vi "FirstCode.vi"() -> ()   [LabVIEW 2015]
uses:
  <vilib>/myRIO/Instrument Drivers/Onboard IO/PWM/typedefs/PWM Reference.ctl
  <vilib>/myRIO/Common/Instrument Driver Framework/Utilities/typedefs/myRIO Generic Hardware Reference.ctl
  <vilib>/myRIO/Common/Instrument Driver Framework/Utilities/typedefs/Hardware Version Enum.ctl
  <vilib>/myRIO/Common/Instrument Driver Framework/Utilities/typedefs/myRIO v1.0 Reference.ctl
  <vilib>/myRIO/Common/Instrument Driver Framework/Utilities/typedefs/Generic FPGA Reference.ctl
  <vilib>/myRIO/Common/Instrument Driver Framework/myRIO v1.0/PWM/typedefs/PWM Channels Enum.ctl
  <vilib>/myRIO/Instrument Drivers/Onboard IO/PWM/typedefs/PWM Configuration.ctl
  <vilib>/userdefined/High Color/nirio_resource_hc.ctl
  <vilib>/myRIO/Instrument Drivers/Onboard IO/DIO/typedefs/DIO Reference.ctl
  <vilib>/myRIO/Common/Instrument Driver Framework/myRIO v1.0/DIO/typedefs/DIO Channels List.ctl
  <vilib>/myRIO/Common/Instrument Driver Framework/myRIO v1.0/DIO/typedefs/DIO Channels Enum.ctl
  <vilib>/myRIO/Common/Instrument Driver Framework/myRIO v1.0/PWM/vis/myRIO v1.1 Open PWM.vi
  <vilib>/myRIO/Common/Instrument Driver Framework/Utilities/vis/Is FPGA Ref Available.vi
  <vilib>/myRIO/Common/Instrument Driver Framework/myRIO v1.0/DIO/vis/myRIO v1.1 Open DIO.vi
  <vilib>/myRIO/Instrument Drivers/Onboard IO/DIO/vis/Read.vi
  <vilib>/myRIO/Instrument Drivers/Onboard IO/DIO/vis/Write.vi
  <vilib>/myRIO/Common/Instrument Driver Framework/Utilities/vis/Validate Channels.vi
  <vilib>/myRIO/Common/Instrument Driver Framework/myRIO v1.0/PWM/vis/myRIO v1.0 Reserve PWM.vi
  <vilib>/myRIO/Instrument Drivers/Onboard IO/PWM/vis/Set Duty Cycle and Frequency.vi
  <vilib>/myRIO/Common/Instrument Driver Framework/myRIO v1.0/DIO/vis/myRIO v1.0 Reserve DIO.vi
  <vilib>/myRIO/Common/Instrument Driver Framework/myRIO v1.0/PWM/vis/myRIO v1.0 Close PWM.vi
  <vilib>/myRIO/Common/Instrument Driver Framework/myRIO v1.0/UART/vis/myRIO v1.0 Close UART.vi
  <vilib>/myRIO/Common/Instrument Driver Framework/myRIO v1.0/PWM/vis/myRIO v1.0 Build MUX Configuration PWM.vi
  <vilib>/myRIO/Common/Instrument Driver Framework/myRIO v1.0/Resource Manager/vis/myRIO v1.0 Reserve Channel List.vi
  <vilib>/myRIO/Common/Instrument Driver Framework/myRIO v1.0/DIO/vis/myRIO v1.0 Build MUX Configuration DIO.vi
  <vilib>/myRIO/Common/Instrument Driver Framework/myRIO v1.0/PWM/vis/myRIO v1.0 Unreserve PWM.vi
  <vilib>/myRIO/Common/Instrument Driver Framework/myRIO v1.0/Resource Manager/vis/myRIO v1.0 Create Configuration List.vi
  <vilib>/myRIO/Common/Instrument Driver Framework/myRIO v1.0/Resource Manager/vis/myRIO v1.0 Reserve Channel.vi
  <vilib>/myRIO/Common/Instrument Driver Framework/myRIO v1.0/Resource Manager/vis/myRIO v1.0 Unreserve Channel.vi
  <vilib>/myRIO/Common/Instrument Driver Framework/myRIO v1.0/Resource Manager/vis/myRIO v1.0 Unreserve Channel List.vi
  <vilib>/myRIO/Common/Instrument Driver Framework/myRIO v1.0/Resource Manager/vis/myRIO v1.0 Build Mutex Name.vi
  <vilib>/Utility/VariantDataType/GetNumericInfo.vi
  <vilib>/Utility/error.llb/Error Cluster From Error Code.vi
  <vilib>/myRIO/Common/Instrument Driver Framework/myRIO v1.0/myRIO v1.1 Open.vi
  <vilib>/myRIO/Common/Instrument Driver Framework/Utilities/vis/IO Manager.vi
  <vilib>/myRIO/Common/Instrument Driver Framework/Utilities/vis/Configuration Manager.vi
  <vilib>/myRIO/Common/Instrument Driver Framework/myRIO v1.0/Resource Manager/vis/myRIO v1.0 Configure IO.vi
  <vilib>/myRIO/Common/Instrument Driver Framework/myRIO v1.0/myRIO v1.0 Close.vi
  <vilib>/myRIO/Common/Instrument Driver Framework/myRIO v1.0/PWM/vis/myRIO v1.0 Write PWM.vi
  <vilib>/myRIO/Common/Instrument Driver Framework/myRIO v1.0/DIO/vis/myRIO v1.0 Write DIO.vi
  <vilib>/myRIO/Common/Instrument Driver Framework/myRIO v1.0/DIO/vis/myRIO v1.0 Read DIO.vi
  <vilib>/myRIO/Common/Instrument Driver Framework/myRIO v1.0/PWM/vis/myRIO v1.0 Shutdown PWM.vi
  <vilib>/myRIO/Common/Instrument Driver Framework/Utilities/vis/FPGA Ref Manager.vi
  <vilib>/myRIO/Common/Instrument Driver Framework/myRIO v1.0/myRIO v1.0 Reset FPGA.vi
  <vilib>/myRIO/Common/Instrument Driver Framework/myRIO v1.0/IRQ/vis/myRIO v1.0 IRQ Info FGV.vi
  <vilib>/myRIO/Common/Instrument Driver Framework/myRIO v1.0/IRQ/vis/myRIO v1.0 Timer IRQ Info FGV.vi
  <vilib>/myRIO/Common/Instrument Driver Framework/myRIO v1.0/IRQ/vis/myRIO v1.0 ISR Agent.vi
  <vilib>/myRIO/Instrument Drivers/Onboard IO/PWM/vis/myRIO PWM Open.xnode
  <vilib>/myRIO/Express VI/Onboard Devices/LED/LED Express VI.xnode
  <vilib>/myRIO/Instrument Drivers/Onboard IO/DIO/vis/myRIO DIO Open.xnode
  <vilib>/myRIO/Express VI/Onboard IO/DI/DI Express VI.xnode
  <vilib>/myRIO/Instrument Drivers/Onboard IO/PWM/PWM.lvlib
  <vilib>/myRIO/Instrument Drivers/Onboard IO/DIO/DIO.lvlib
  <vilib>/myRIO/Instrument Drivers/Utilities/Utilities.lvlib
panel:
  out "Sensor Pin":T1
  out "Gripper Pin":T1
  out "Pour Pin":T1
  in  "Pour":bool
  out "Information":string="Pour"
  out "Counter":dbl=1.0
  out "New Duty Cycle":dbl=nan
  in  "Stop [ESC]":bool
  in  "Sensor":bool
  in  "Gripper":bool
  out "Water Detected":bool
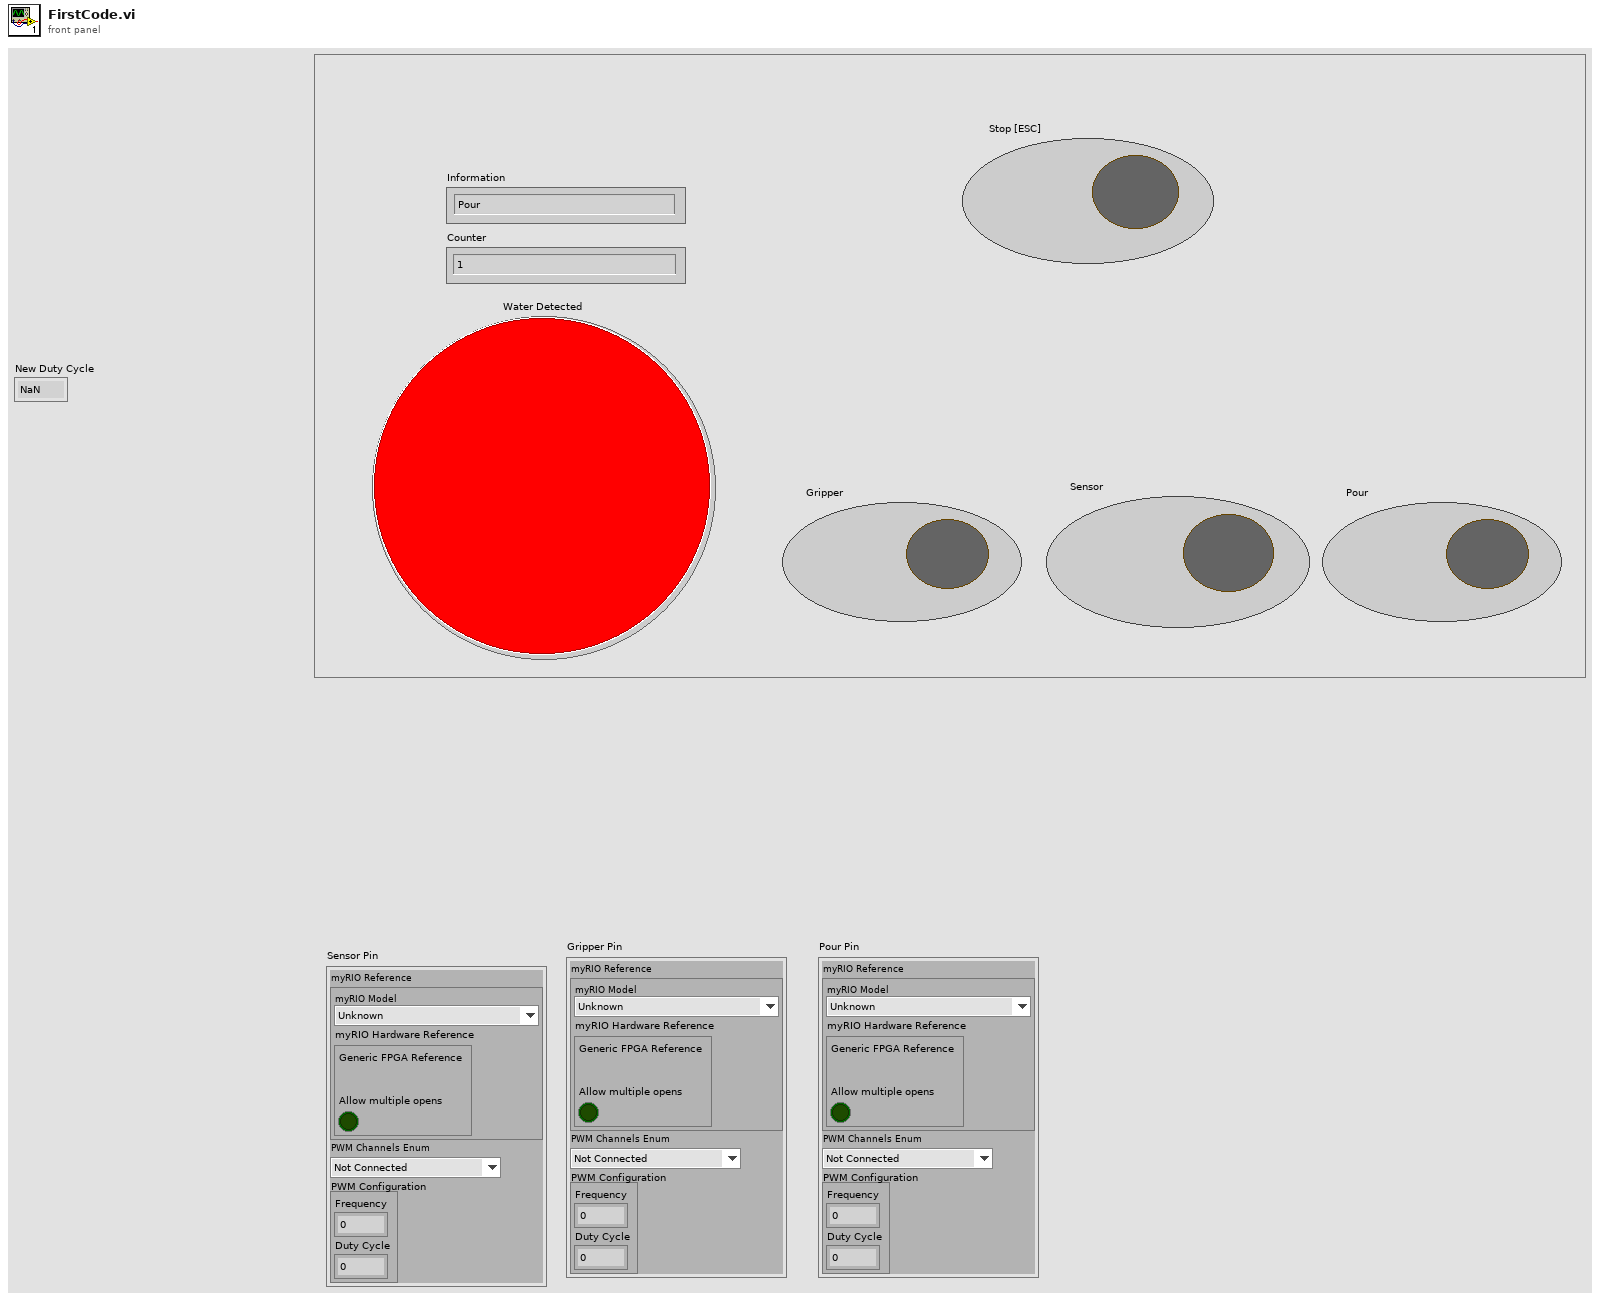
[diagram p1: front panel]
types:
  T1 = typedef "PWM.lvlib/PWM Reference.ctl" = cluster{"myRIO Reference":T2, "PWM Channels Enum":T6, "PWM Configuration":T7}
  T2 = typedef "myRIO Generic Hardware Reference.ctl" = cluster{"myRIO Model":T3, "myRIO Hardware Reference":T4}
  T3 = typedef "Hardware Version Enum.ctl" = enum16{"Unknown", "myRIO-1900", "myRIO-1950", "roboRIO"}
  T4 = typedef "myRIO v1.0 Reference.ctl" = cluster{"Generic FPGA Reference":T5, "Allow multiple opens":bool}
  T5 = typedef "Generic FPGA Reference.ctl" = refnum<k20>
  T6 = typedef "PWM Channels Enum.ctl" = enum16{"Not Connected", "C/PWM0", "C/PWM1", "A/PWM0", "A/PWM1", "A/PWM2", "B/PWM0", "B/PWM1", "B/PWM2", "PWM/PWM0", "PWM/PWM1", "PWM/PWM2", "PWM/PWM3", "PWM/PWM4", "PWM/PWM5", "PWM/PWM6", "PWM/PWM7", "PWM/PWM8", "PWM/PWM9"}
  T7 = typedef "PWM.lvlib/PWM Configuration.ctl" = cluster{"Frequency":dbl, "Duty Cycle":dbl}
  T8 = typedef "nirio_resource_hc.ctl" = tag
  T9 = typedef "DIO.lvlib/DIO Reference.ctl" = cluster{"myRIO Reference":T2, "DIO Channels List":T10}
  T10 = typedef "DIO Channels List.ctl" = T11[]
  T11 = typedef "DIO Channels Enum.ctl" = enum16{"Not Connected", "C/DIO0", "C/DIO1", "C/DIO2", "C/DIO3", "C/DIO4", "C/DIO5", "C/DIO6", "C/DIO7", "A/DIO0", "A/DIO1", "A/DIO2", "A/DIO3", "A/DIO4", "A/DIO5", "A/DIO6", "A/DIO7", "A/DIO8", "A/DIO9", "A/DIO10", "A/DIO11", "A/DIO12", "A/DIO13", "A/DIO14", "A/DIO15", "B/DIO0", "B/DIO1", "B/DIO2", "B/DIO3", "B/DIO4", "B/DIO5", "B/DIO6", "B/DIO7", "B/DIO8", "B/DIO9", "B/DIO10", "B/DIO11", "B/DIO12", "B/DIO13", "B/DIO14", "B/DIO15", "LED0", "LED1", "LED2", "LED3", "Button0", "DIO/DIO0", "DIO/DIO1", "DIO/DIO2", "DIO/DIO3", "DIO/DIO4", "DIO/DIO5", "DIO/DIO6", "DIO/DIO7", "DIO/DIO8", "DIO/DIO9", "SPI/CS0", "SPI/CS1", "SPI/CS2", "SPI/CS3", "LED RADIO (Green)", "LED RADIO (Red)", "LED COMM (Green)", "LED COMM (Red)", "LED MODE (Green)", "LED MODE (Red)"}
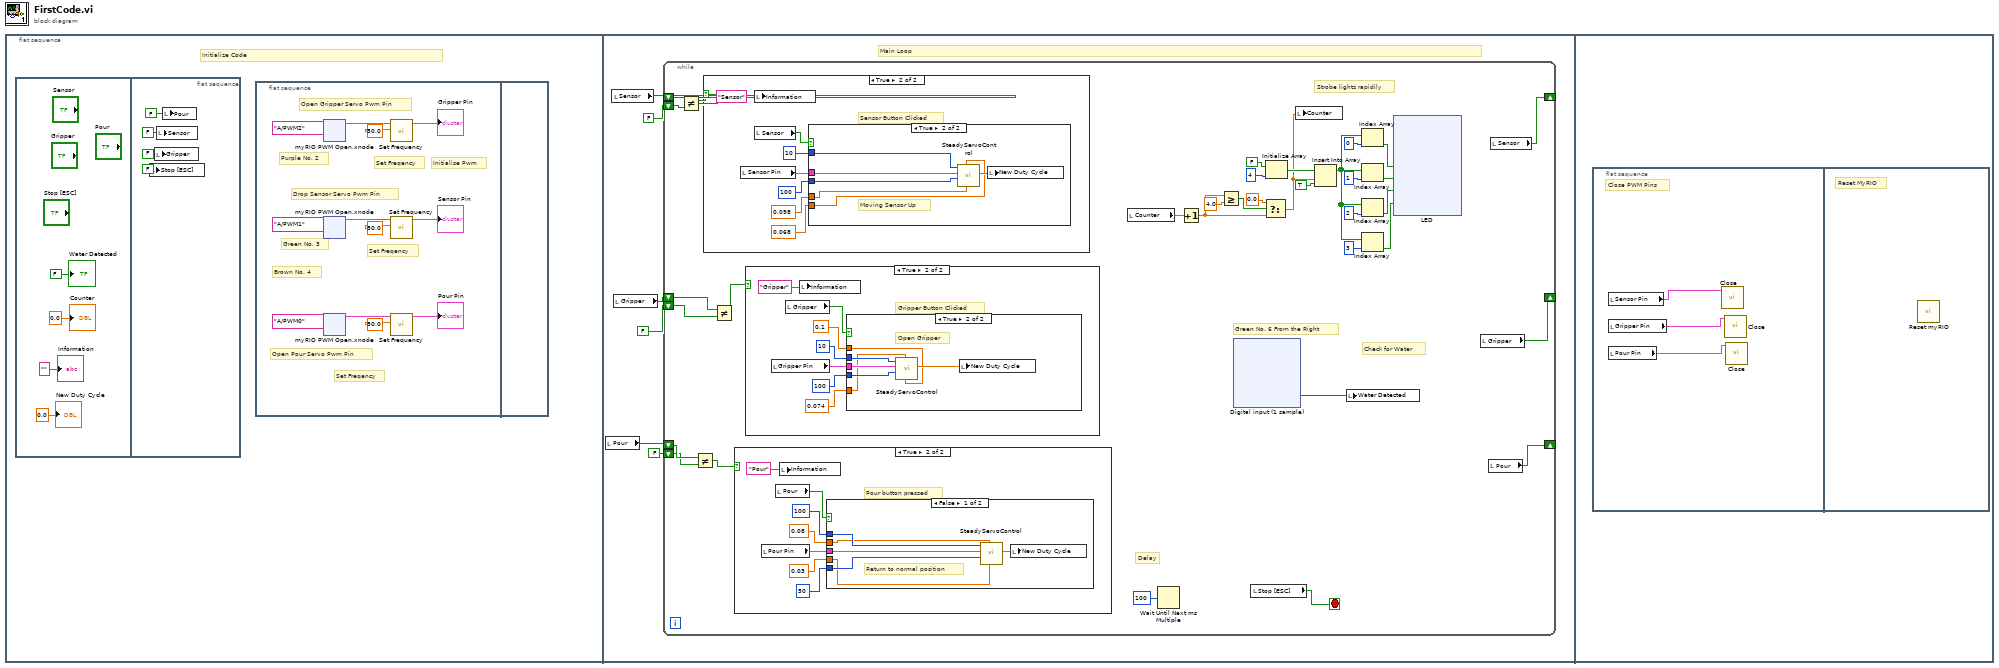
[diagram p0: block diagram]
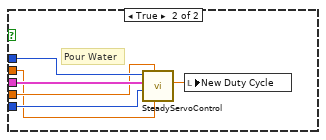
[diagram p3: hidden frame]
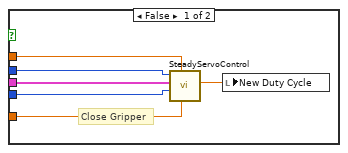
[diagram p5: hidden frame]
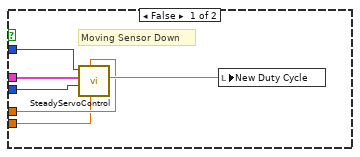
[diagram p7: hidden frame]
diagram:
  n1 = flat-sequence {
    frame #0 {
      # "Initialize Code"
      n2 = flat-sequence {
        frame #0 {
          "Water Detected" <- FALSE ("Water Detected")
          "Counter" <- 0.0 ("Counter")
          "Information" <- "" ("Information")
          "New Duty Cycle" <- 0.0 ("New Duty Cycle")
        }
        frame #1 {
          n3 = local write "Stop [ESC]"(FALSE ("Pour")) -> ()
          n4 = local write "Gripper"(FALSE ("Pour")) -> ()
          n5 = local write "Sensor"(FALSE ("Pour")) -> ()
          n6 = local write "Pour"(FALSE ("Pour")) -> ()
        }
      }
      n7 = flat-sequence {
        frame #0 {
          # "Green No. 3"
          # "Set Freqency"
          # "Drop Sensor Servo Pwm Pin"
          # "Initialise Pwm"
          # "Purple No. 2"
          # "Set Freqency"
          # "Open Gripper Servo Pwm Pin"
          # "Set Freqency"
          # "Brown No. 4"
          # "Open Pour Servo Pwm Pin"
          n8 = xnode "myRIO PWM Open.xnode"("Channel Name"=tag "A/PWM2") -> ("PWM Ref Out"=w7:T1)  [unwired: 2 in, 1 out]
          n9 = xnode "myRIO PWM Open.xnode"("Channel Name"=tag "A/PWM1") -> ("PWM Ref Out"=w2:T1)  [unwired: 2 in, 1 out]
          n10 = xnode "myRIO PWM Open.xnode"("Channel Name"=tag "A/PWM0") -> ("PWM Ref Out"=w10:T1)  [unwired: 2 in, 1 out]
          n11 = call <vilib>:"Set Frequency.vi"("Frequency [Hz]"=50.0, "PWM Ref In"=w7) -> ("PWM Ref Out"=→"Gripper Pin":T1)  [unwired: 7 in, 1 out]
          n12 = call <vilib>:"Set Frequency.vi"("Frequency [Hz]"=50.0, "PWM Ref In"=w2) -> ("PWM Ref Out"=→"Sensor Pin":T1)  [unwired: 7 in, 1 out]
          n13 = call <vilib>:"Set Frequency.vi"("Frequency [Hz]"=50.0, "PWM Ref In"=w10) -> ("PWM Ref Out"=→"Pour Pin":T1)  [unwired: 7 in, 1 out]
        }
        frame #1 {
        }
      }
    }
    frame #1 {
      # "Main Loop"
      n14 = local read "Pour"() -> (w70:bool)
      n15 = local read "Sensor"() -> (w74:bool)
      n16 = local read "Gripper"() -> (w72:bool)
      n17 = while {
        shift-right: [w108] -> _
        shift-left: w74 -> [w75]
        shift-left: FALSE ("Sensor") -> [w107]
        shift-right: [w105] -> _
        shift-left: w72 -> [w103]
        shift-left: FALSE ("Gripper") -> [w102]
        shift-right: [w76] -> _
        shift-left: w70 -> [w78]
        shift-left: FALSE ("Pour") -> [w77]
        stop <- w101 stop-if-true
        # "Delay"
        # "Check for Water"
        # "Strobe lights rapidily"
        # "Green No. 6 From the Right"
        n18 = Not Equal?(x=w75, y=w107) -> (x != y?=w106:bool)
        n19 = Not Equal?(x=w78, y=w77) -> (x != y?=w79:bool)
        n20 = case shown="True" w106 {
          frame False {
          }
          frame True {
            # "Sensor Button Clicked"
            n21 = local read "Sensor Pin"() -> (w222:T1)
            n22 = local write "Information"("Sensor" ("Information")) -> ()
            n23 = local read "Sensor"() -> (w225:bool)
            n24 = case shown="True" w225 {
              tunnel: u32 10 ("Wait Time") -> [w230 w237]
              tunnel: 100 ("Steps") -> [w229 w236]
              tunnel: w222 -> [w231 w235]
              tunnel: 0.098 ("t") -> [w228 w233]
              tunnel: 0.068 ("f") -> [w227 w234]
              frame False {
                # "Moving Sensor Down"
                n25 = call "SteadyServoControl.vi"("New Duty Cycle"=w227, "Prev Duty Cycle"=w228, "Steps"=w229, "PWM Ref Out in"=w231, "Wait Time"=w230) -> ("Numeric"=w232:dbl)  [unwired: 5 in, 1 out]
                n26 = local write "New Duty Cycle"(w232) -> ()
              }
              frame True {
                # "Moving Sensor Up"
                n27 = call "SteadyServoControl.vi"("New Duty Cycle"=w233, "Prev Duty Cycle"=w234, "Steps"=w236, "PWM Ref Out in"=w235, "Wait Time"=w237) -> ("Numeric"=w238:dbl)  [unwired: 5 in, 1 out]
                n28 = local write "New Duty Cycle"(w238) -> ()
              }
            }
          }
        }
        n29 = Not Equal?(x=w103, y=w102) -> (x != y?=w104:bool)
        n30 = case shown="True" w79 {
          frame False {
          }
          frame True {
            # "Pour button pressed"
            n31 = local read "Pour Pin"() -> (w113:T1)
            n32 = local read "Pour"() -> (w114:bool)
            n33 = local write "Information"("Pour" ("Information")) -> ()
            n34 = case shown="False" w114 {
              tunnel: w113 -> [w120 w127]
              tunnel: 50 ("Steps") -> [w118 w125]
              tunnel: u32 100 ("Wait Time") -> [w119 w124]
              tunnel: 0.03 ("Prev Duty Cycle") -> [w117 w123]
              tunnel: 0.08 ("New Duty Cycle") -> [w116 w122]
              frame False {
                # "Return to normal position"
                n35 = call "SteadyServoControl.vi"("New Duty Cycle"=w117, "Prev Duty Cycle"=w116, "Steps"=w118, "PWM Ref Out in"=w120, "Wait Time"=w119) -> ("Numeric"=w121:dbl)  [unwired: 5 in, 1 out]
                n36 = local write "New Duty Cycle"(w121) -> ()
              }
              frame True {
                # "Pour Water"
                n37 = call "SteadyServoControl.vi"("New Duty Cycle"=w122, "Prev Duty Cycle"=w123, "Steps"=w125, "PWM Ref Out in"=w127, "Wait Time"=w124) -> ("Numeric"=w126:dbl)  [unwired: 5 in, 1 out]
                n38 = local write "New Duty Cycle"(w126) -> ()
              }
            }
          }
        }
        n39 = case shown="True" w104 {
          frame False {
          }
          frame True {
            # "Gripper Button Clicked"
            n40 = local read "Gripper Pin"() -> (w205:T1)
            n41 = local read "Gripper"() -> (w206:bool)
            n42 = local write "Information"("Gripper" ("Information")) -> ()
            n43 = case shown="True" w206 {
              tunnel: w205 -> [w212 w216]
              tunnel: u32 10 ("Wait Time") -> [w211 w218]
              tunnel: 100 ("Steps") -> [w210 w217]
              tunnel: 0.074 ("Prev Duty Cycle") -> [w209 w215]
              tunnel: 0.1 ("New Duty Cycle") -> [w208 w214]
              frame False {
                # "Close Gripper"
                n44 = call "SteadyServoControl.vi"("New Duty Cycle"=w209, "Prev Duty Cycle"=w208, "Steps"=w210, "PWM Ref Out in"=w212, "Wait Time"=w211) -> ("Numeric"=w213:dbl)  [unwired: 5 in, 1 out]
                n45 = local write "New Duty Cycle"(w213) -> ()
              }
              frame True {
                # "Open Gripper"
                n46 = call "SteadyServoControl.vi"("New Duty Cycle"=w214, "Prev Duty Cycle"=w215, "Steps"=w217, "PWM Ref Out in"=w216, "Wait Time"=w218) -> ("Numeric"=w219:dbl)  [unwired: 5 in, 1 out]
                n47 = local write "New Duty Cycle"(w219) -> ()
              }
            }
          }
        }
        n48 = local read "Counter"() -> (w80:dbl)
        n49 = Wait Until Next ms Multiple(millisecond multiple=u32 100) -> ()  [unwired: 1 out]
        n50 = Increment(x=w80) -> (x+1=w95:dbl)
        n51 = Greater Or Equal?(x=w95, y=4.0) -> (x >= y?=w97:bool)
        n52 = xnode "Digital input (1 sample)"() -> ("A/DIO0 (Pin 11)"=w100:bool)  [unwired: 1 in, 1 out]
        n53 = local read "Stop [ESC]"() -> (w101:bool)
        n54 = Select(t=0.0, s=w97, f=w95) -> (s? t:f=w81:dbl)
        n55 = Initialize Array(FALSE, 4 ("dimension size")) -> (w84:bool[])
        n56 = local write "Counter"(w81) -> ()
        n57 = Insert Into Array(array=w84, index=w81, new element=TRUE ("new element/subarray")) -> (w83:bool[])
        n58 = local write "Water Detected"(w100) -> ()
        n59 = Index Array(array=w83, index=0) -> (element=w93:bool)
        n60 = Index Array(array=w83, index=1) -> (element=w87:bool)
        n61 = Index Array(array=w83, index=2) -> (element=w86:bool)
        n62 = Index Array(array=w83, index=3) -> (element=w85:bool)
        n63 = xnode "LED"("LED0"=w93, "LED1"=w87, "LED2"=w86, "LED3"=w85) -> ()  [unwired: 1 in, 1 out]
        n64 = local read "Gripper"() -> (w105:bool)
        n65 = local read "Pour"() -> (w76:bool)
        n66 = local read "Sensor"() -> (w108:bool)
      }
    }
    frame #2 {
      n67 = flat-sequence {
        frame #0 {
          # "Close PWM Pins"
          n68 = local read "Sensor Pin"() -> (w239:T1)
          n69 = local read "Gripper Pin"() -> (w240:T1)
          n70 = local read "Pour Pin"() -> (w241:T1)
          n71 = call <vilib>:"Close.vi"("PWM Ref In"=w239) -> ()  [unwired: 10 in, 1 out]
          n72 = call <vilib>:"Close.vi"("PWM Ref In"=w240) -> ()  [unwired: 10 in, 1 out]
          n73 = call <vilib>:"Close.vi"("PWM Ref In"=w241) -> ()  [unwired: 10 in, 1 out]
        }
        frame #1 {
          # "Reset MyRIO"
          n74 = call <vilib>:"Reset myRIO.vi"() -> ()  [unwired: 11 in, 1 out]
        }
      }
    }
  }
